vi "TW Replace Missing Dependency VIs - Client Wrapper.vi"(8 "error in":errorcluster, 10 "gRPC Service Name":string, 11 "Project Path":path) -> (0 "error out":errorcluster)   [LabVIEW 2021, in "Plugin Generator.lvlib"]
uses:
  Plugin Generator.lvlib
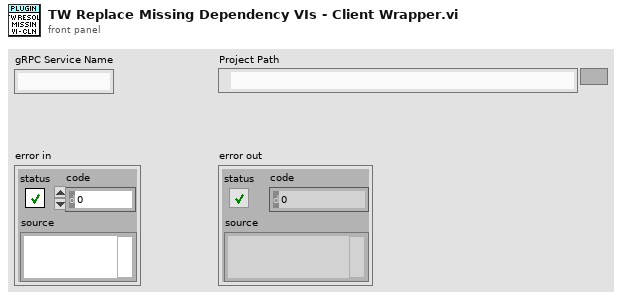
[diagram p1: front panel]
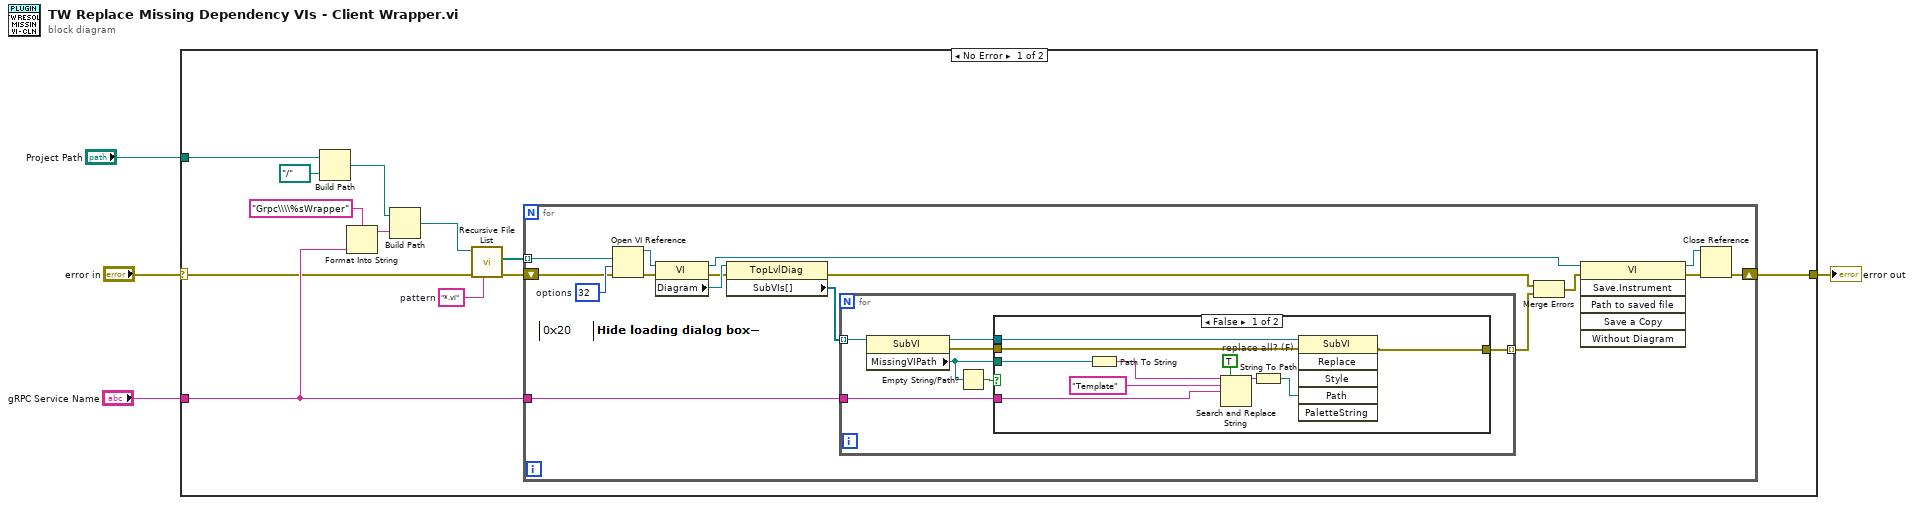
[diagram p0: block diagram]
diagram:
  n1 = case shown="No Error" "error in" {
    selector: "error in" -> [w9 w51]
    tunnel: [w8 w51] -> w4
    tunnel: "gRPC Service Name" -> [w11 _]
    tunnel: "Project Path" -> [w6 _]
    frame No Error {
      w15 = "*.vi"  # pattern
      n2 = Build Path(base path=w6, name or relative path=path "../..") -> (appended path=w5:path)
      n3 = Format Into String(format string="Grpc\\\\%sWrapper" ("Class Name"), w11) -> (resulting string=w14:string)  [unwired: 2 in, 1 out]
      n4 = Build Path(base path=w5, name or relative path=w14) -> (appended path=w13:path)
      n5 = call <vilib>:"Recursive File List.vi"("pattern"=w15, "error in (no error)"=w9, "Folder Path"=w13) -> ("error out"=w10:errorcluster, "All Files in Dir"=w16:path[])  [unwired: 4 in, 3 out]
      n6 = for {
        tunnel: w16 -> [w32] mode=indexing
        tunnel: w11 -> [w27]
        shift-right: [w24] -> w8
        shift-left: w10 -> [w22]
        w23 = 32  # options
        n7 = Open VI Reference(vi path=w32, options=w23, error in (no error)=w22) -> (vi reference=w31:refnum<vi>, error out=w25:errorcluster)  [unwired: 3 in]
        n8 = property class="VI"(reference=w31, error in=w25) -> (reference out=w29:refnum<vi>, error out=w26:errorcluster, "Diagram"=w30:refnum<vi>)
        n9 = property class="TopLvlDiag"(reference=w30, error in=w26) -> (error out=w17:errorcluster, "SubVIs[]"=w28:refnum<vi>[])  [unwired: 1 out]
        n10 = for {
          tunnel: w28 -> [w39] mode=indexing
          tunnel: w27 -> [w35]
          tunnel: [w33] -> w18 mode=indexing
          n11 = property class="SubVI"(reference=w39) -> (reference out=w37:refnum<vi>, error out=w34:errorcluster, "MissingVIPath"=w36:path)  [unwired: 1 in]
          n12 = Empty String/Path?(string/path=w36) -> (empty?=w38:bool)
          n13 = case shown="False" w38 {
            tunnel: w37 -> [w49 _]
            tunnel: w36 -> [w47 _]
            tunnel: w35 -> [w43 _]
            tunnel: w34 -> [w41 w50]
            tunnel: [w40 w50] -> w33
            frame False {
              w42 = TRUE  # replace all? (F)
              n14 = Path To String(path=w47) -> (string=w48:string)
              n15 = Search and Replace String(replace all?=w42, input string=w48, search string="Template", replace string=w43) -> (result string=w45:string)  [unwired: 4 in, 3 out]
              n16 = String To Path(string=w45) -> (path=w44:path)
              n17 = invoke class="SubVI" method="Replace"(reference=w49, error in=w41, "Path"=w44) -> (error out=w40:errorcluster)  [unwired: 3 in, 5 out]
            }
            frame True {
            }
          }
        }
        n18 = Merge Errors(w17, w18) -> (w19:errorcluster)
        n19 = invoke class="VI" method="Save.Instrument"(reference=w29, error in=w19) -> (reference out=w21:refnum<vi>, error out=w20:errorcluster)  [unwired: 4 in, 4 out]
        n20 = Close Reference(reference=w21, error in (no error)=w20) -> (error out=w24:errorcluster)
      }
    }
    frame Error {
    }
  }
  "error out" <- w4
